vi "电导率_所有参数读取.vi"(8 "error in (no error)":errorcluster caption="错误输入（无错误）", 11 "MB_Serial session in":refnum<class "MB_Master_Serial.lvclass">) -> (0 "error out":errorcluster caption="错误输出", 2 "输出值":T1 {"电极型号标志" items=["NULL", "pH", "Cond", "DO", "Turb"]; "电极状态标志" items=["OK"]}, 3 "MB_Serial session out":refnum<class "MB_Master_Serial.lvclass">)   [LabVIEW 2016, in "斯坦道多参数.lvlib"]
uses:
  <vilib>/Plasmionique/MB Master/MB_Master_Serial/MB_Master_Serial.lvclass
  C:/Program Files (x86)/National Instruments/LabVIEW 2016/vi.lib/Plasmionique/MB Master/MB_Master/MB_Master.lvclass
  <vilib>/Plasmionique/MB Master/MB Master.lvlib
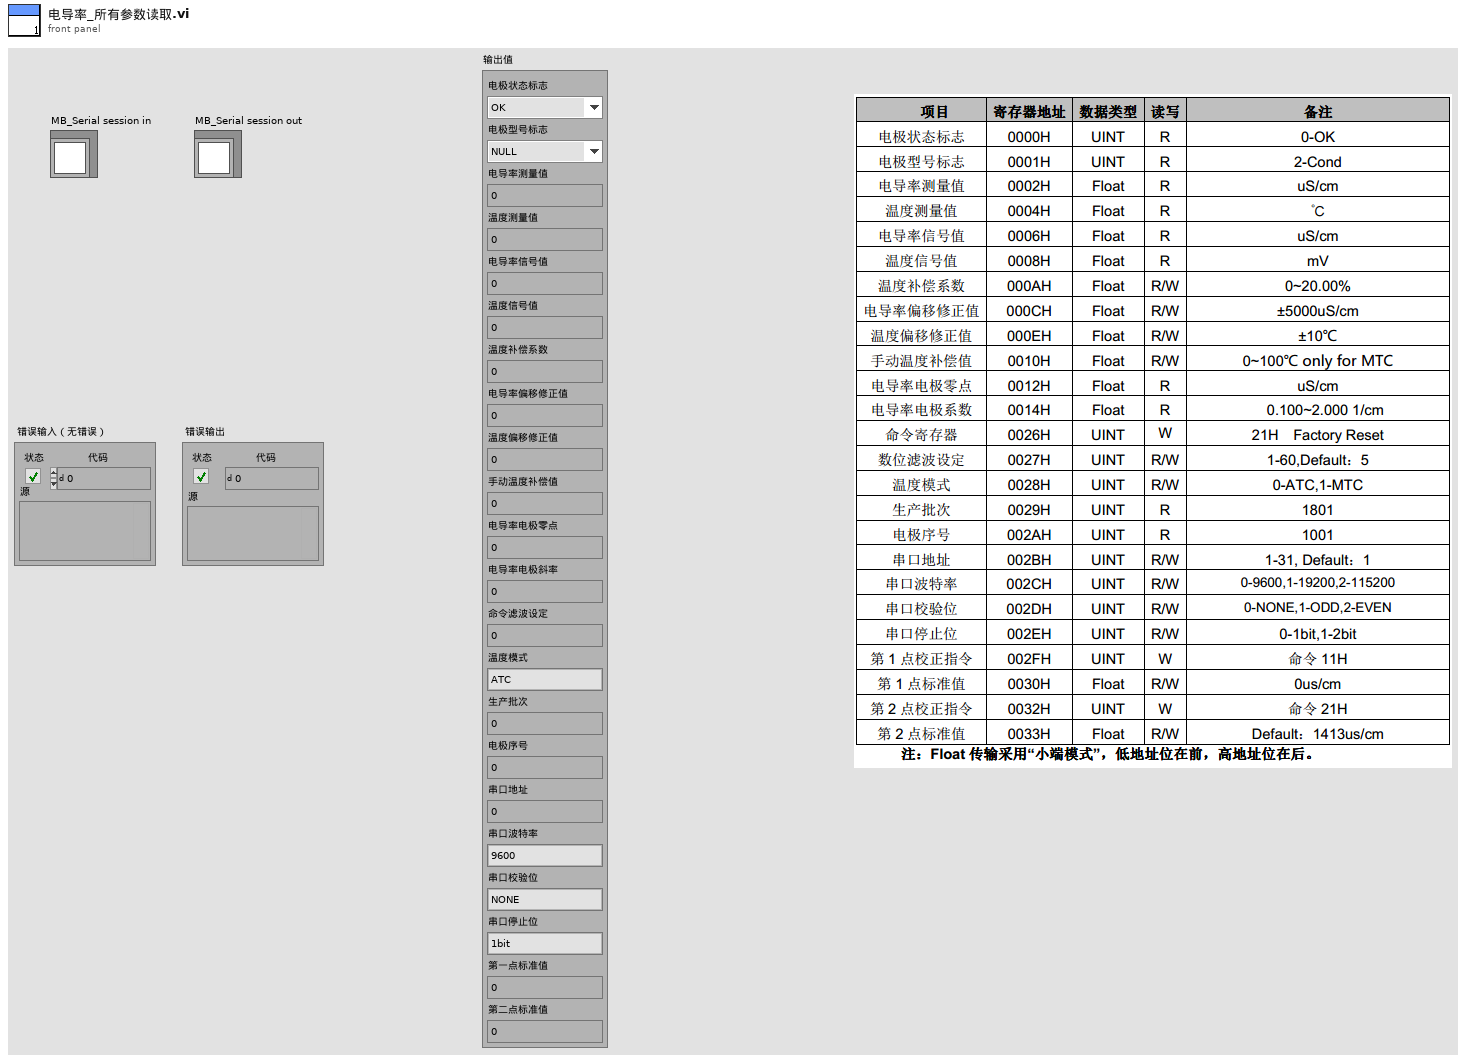
[diagram p1: front panel]
types:
  T1 = cluster{"电极状态标志":u16, "电极型号标志":u16, "电导率测量值":sgl, "温度测量值":sgl, "电导率信号值":sgl, "温度信号值":sgl, "温度补偿系数":sgl, "电导率偏移修正值":sgl, "温度偏移修正值":sgl, "手动温度补偿值":sgl, "电导率电极零点":sgl, "电导率电极斜率":sgl, "命令滤波设定":u16, "温度模式":enum16{"ATC", "MTC"}, "生产批次":u16, "电极序号":u16, "串口地址":u16, "串口波特率":enum16{"9600", "19200", "115200"}, "串口校验位":enum16{"NONE", "ODD", "EVEN"}, "串口停止位":enum16{"1bit", "2bit"}, "第一点标准值":sgl, "第二点标准值":sgl}
  T2 = cluster{u16, u16, "数值":sgl, "数值":sgl, "数值":sgl, "数值":sgl, "数值":sgl, "数值":sgl, "数值":sgl, "数值":sgl, "数值":sgl, "数值":sgl, u16, u16, u16, u16, u16, u16, u16, u16, "数值":sgl, "数值":sgl}
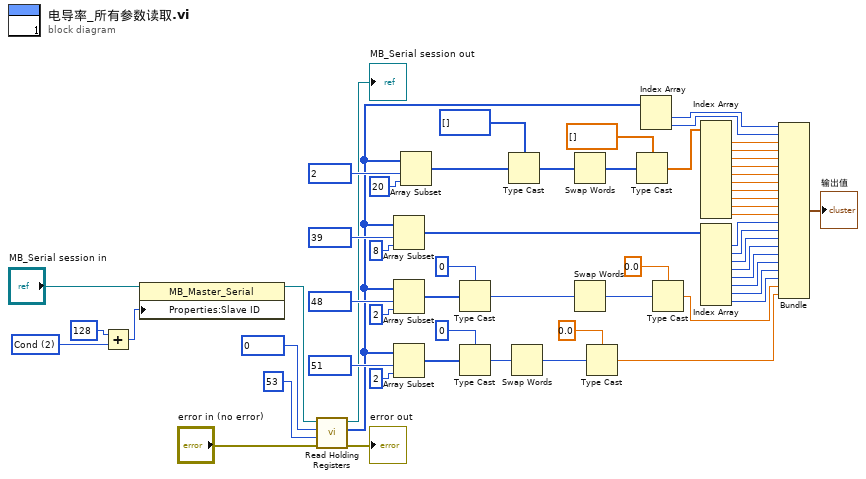
[diagram p0: block diagram]
diagram:
  w59 = u16 2 items=["NULL", "pH", "Cond", "DO", "Turb"] ("数值")
  n1 = Add(x=u16 128, y=w59) -> (x+y=w57:u16)
  n2 = property class="MB_Master_Serial"(reference="MB_Serial session in", "Properties:Slave ID"=w57) -> (reference out=w9:refnum<class "MB_Master_Serial.lvclass">)  [unwired: 1 in, 1 out]
  n3 = call <vilib>:"Read Holding Registers.vi"("error in (no error)"="error in (no error)", "quantity"=u16 53, "starting address"=u16 0, "MB session in"=w9) -> ("error out"=→"error out":errorcluster, "Registers"=w24:u16[], "MB session out"=→"MB_Serial session out":refnum<class "MB_Master_Serial.lvclass">)  [unwired: 5 in]
  n4 = Array Subset(array=w24, index=u16 39 ("starting address"), length=8 ("长度")) -> (w37:u16[])
  n5 = Array Subset(array=w24, index=u16 48 ("starting address"), length=2 ("长度")) -> (w19:u16[])
  n6 = Array Subset(array=w24, index=u16 51 ("starting address"), length=2 ("长度")) -> (w14:u16[])
  n7 = Array Subset(array=w24, index=u16 2 ("starting address"), length=20 ("长度")) -> (w46:u16[])
  n8 = Type Cast(type=u32 0 ("数值"), x=w19) -> (*(type *) &x=w22:u32)
  n9 = Type Cast(type=u32 0 ("数值"), x=w14) -> (*(type *) &x=w16:u32)
  n10 = Type Cast(type=u32[] [] ("数组 2"), x=w46) -> (*(type *) &x=w48:u32[])
  n11 = Swap Words(1:w16) -> (0:w15:u32)
  n12 = Swap Words(1:w48) -> (0:w50:u32[])
  n13 = Swap Words(1:w22) -> (0:w23:u32)
  n14 = Type Cast(type=sgl 0.0 ("数值"), x=w15) -> (*(type *) &x=w12:sgl)
  n15 = Type Cast(type=sgl[] [] ("数组 2"), x=w50) -> (*(type *) &x=w45:sgl[])
  n16 = Index Array(array=w24) -> (element #1=w53:u16, element #2=w52:u16)  [unwired: 2 in]
  n17 = Type Cast(type=sgl 0.0 ("数值"), x=w23) -> (*(type *) &x=w13:sgl)
  n18 = Index Array(array=w45) -> (element #1=w44:sgl, element #2=w43:sgl, element #3=w42:sgl, element #4=w41:sgl, element #5=w7:sgl, element #6=w6:sgl, element #7=w5:sgl, element #8=w4:sgl, element #9=w3:sgl, element #10=w2:sgl)  [unwired: 10 in]
  n19 = Index Array(array=w37) -> (element #1=w36:u16, element #2=w35:u16, element #3=w34:u16, element #4=w33:u16, element #5=w32:u16, element #6=w31:u16, element #7=w30:u16, element #8=w29:u16)  [unwired: 8 in]
  n20 = Bundle(w53, w52, "数值"=w44, "数值"=w43, "数值"=w42, "数值"=w41, "数值"=w7, "数值"=w6, "数值"=w5, "数值"=w4, "数值"=w3, "数值"=w2, w36, w35, w34, w33, w32, w31, w30, w29, "数值"=w13, "数值"=w12) -> (→"输出值":T2)  [unwired: 1 in]
